vi "Create.vi"(8 "error in":errorcluster) -> (0 "error out":errorcluster, 3 "Potting Procedure out":refnum<class "Potting Procedure.lvclass">)   [LabVIEW 2011, in "Potting Procedure.lvclass"]
uses:
  Potting Procedure.lvclass
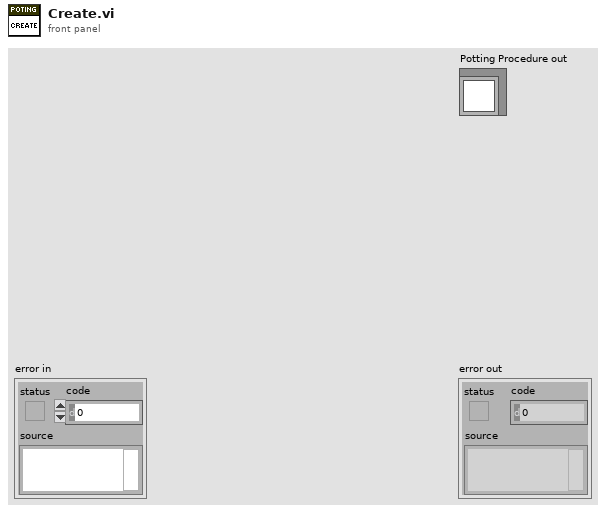
[diagram p1: front panel]
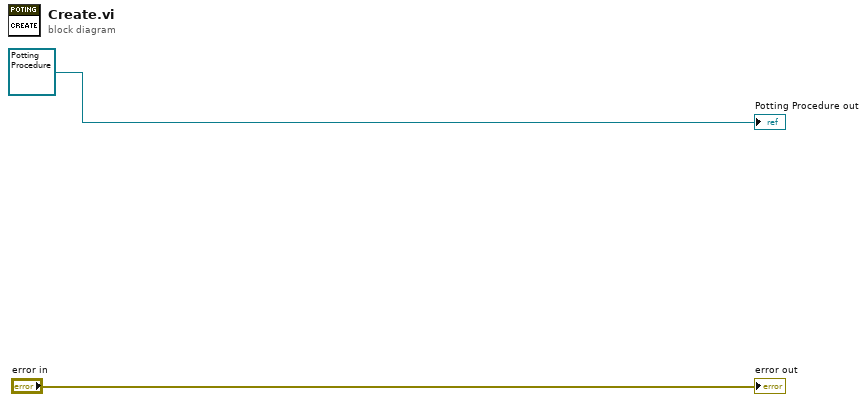
[diagram p0: block diagram]
diagram:
  "error out" <- "error in"
  "Potting Procedure out" <- refnum<class "Potting Procedure.lvclass"> refnum ("Potting Procedure in")
